vi "计算散斑矩阵列平均值.vi"(1 "散斑二维数组":dbl[][](array[numeric]), 2 "散斑二维数组行数":i32) -> (0 "散斑二维数组列平均值":dbl[](array[numeric]))   [LabVIEW 2018]
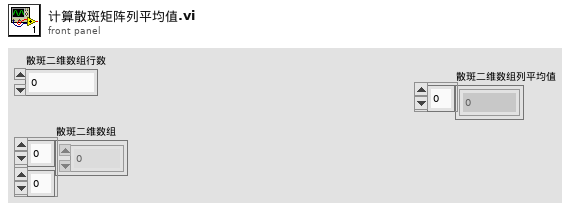
[diagram p1: front panel]
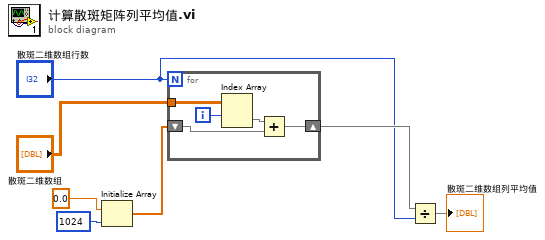
[diagram p0: block diagram]
diagram:
  n1 = Initialize Array(0.0, 1024) -> (w5:dbl[])
  n2 = for {
    N: "散斑二维数组行数" -> [_]
    shift-right: [w8] -> w7
    shift-left: w5 -> [w9]
    tunnel: "散斑二维数组" -> [w12]
    i -> [w11]
    n3 = Index Array(array=w12, index (row)=w11) -> (element=w10:dbl[])  [unwired: 1 in]
    n4 = Add(x=w10, y=w9) -> (x+y=w8:dbl[])
  }
  n5 = Divide(x=w7, y="散斑二维数组行数") -> (x/y=→"散斑二维数组列平均值":dbl[])
